vi "Install Set.vi"(7 "Restart Automatically (T)":bool=TRUE, 8 "error in (no error)":errorcluster, 9 "Add-ons to Install":T1[](array[typedef]) {"component type" items=["standard", "hidden", "system", "unknown", "startup", "image"]}, 10 "Software Set":T1 {"component type" items=["standard", "hidden", "system", "unknown", "startup", "image"]}, 11 "Session in":refnum<k21>) -> (0 "error out":errorcluster, 1 "Broken Dependencies":T3[](array[typedef]) {"dependee"."component type" items=["standard", "hidden", "system", "unknown", "startup", "image"]; "depender"."component type" items=["standard", "hidden", "system", "unknown", "startup", "image"]}, 3 "Session out":refnum<k21>)   [LabVIEW 2014, in "nisyscfg.lvlib"]
doc: "Use the Install Set VI to install all included components in the software set, even if the component is already installed on the target, and uninstall currently installed components that are not part of the software set."
uses:
  nisyscfg.lvlib
  Software 1.2.ctl
  Component Type.ctl
  Broken Dependency 1.2.ctl
  Error Cluster From Error Code.vi
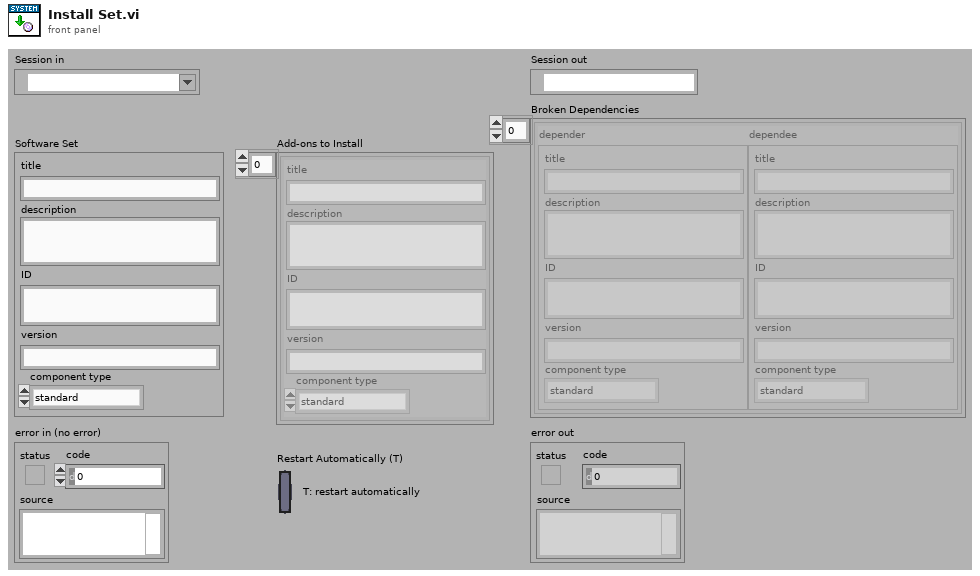
[diagram p1: front panel]
types:
  T1 = typedef "nisyscfg.lvlib/Software 1.2.ctl" = cluster{"title":string, "description":string, "ID":string, "version":string, "component type":T2}
  T2 = typedef "nisyscfg.lvlib/Component Type.ctl" = u32
  T3 = typedef "nisyscfg.lvlib/Broken Dependency 1.2.ctl" = cluster{"depender":T1, "dependee":T1}
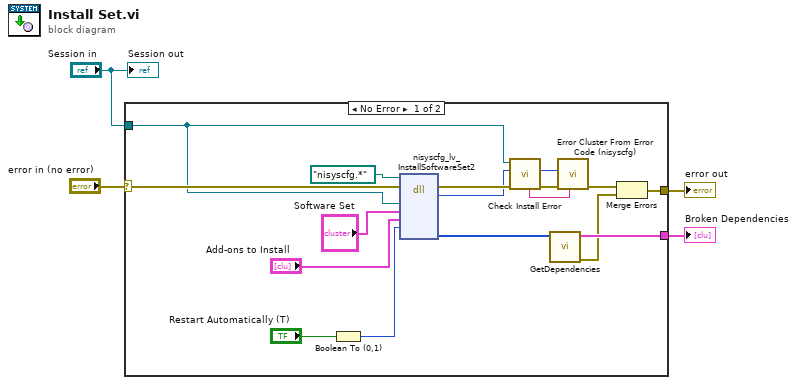
[diagram p0: block diagram]
diagram:
  n1 = case shown="No Error" "error in (no error)" {
    selector: "error in (no error)" -> [w16 w22]
    tunnel: "Session in" -> [w10 _]
    tunnel: [w19 _] -> w4
    tunnel: [w15 w22] -> w2
    frame No Error {
      n2 = Boolean To (0,1)(Boolean="Restart Automatically (T)") -> (0, 1=w13:i16)
      n3 = dll-call lib="nisyscfg.*" fn="nisyscfg_lv_InstallSoftwareSet2" label="InstallSoftwareSet"(path in=path "nisyscfg.*", error in=w16, "system"=w10, "softwareSetInfo"="Software Set", "addOns"="Add-ons to Install", "restartAutomatically"=w13) -> (error out=w9:errorcluster, "result"=w8:i32, "brokenDependencies"=w20:u64[])  [unwired: 6 in, 1 out]
      n4 = call "Check Install Error.vi"("error in (no error)"=w9, "Status in"=w8, "Session in"=w10) -> ("error out"=w11:errorcluster, "Status out"=w6:i32, "Details"=w5:string)  [unwired: 5 in, 1 out]
      n5 = call "GetDependencies.vi"("Enumerator in"=w20) -> ("error out"=w17:errorcluster, "Dependencies"=w19:T3[])  [unwired: 9 in]
      n6 = call "Error Cluster From Error Code (nisyscfg).vi"("Details String"=w5, "error in (no error)"=w11, "Error Code (0)"=w6) -> ("error out"=w7:errorcluster)  [unwired: 8 in]
      n7 = Merge Errors(w7, w17) -> (w15:errorcluster)
    }
    frame Error {
    }
  }
  "error out" <- w2
  "Broken Dependencies" <- w4
  "Session out" <- "Session in"
